vi "Query to Tree Information.vi"(7 "System or ALL Combined Fields":T1[](array[typedef]), 8 "error in (no error)":errorcluster, 9 "Load data? (t)":bool=TRUE, 10 "Load Fields? (f)":bool, 11 "Run Array":T9[](array[typedef])) -> (0 "error out":errorcluster, 1 "Total ms":u32, 3 "Data Tree":T4[](array[typedef]))   [LabVIEW 2011]
uses:
  www/cgi-bin/_cgi-lib/TDM_INDEX Record.ctl
  TDMS/TDMS Model Number.ctl
  TDMS/TDMS Serial Number.ctl
  TDMS/TDMS File.ctl
  TDMS/TDMS Run.ctl
  TDMS/TDMS Channel (Sxx).ctl
  database/Fields/Field Record.ctl
  database/Fields/Field DataTypes.ctl
  database/Fields/Field NextItem.ctl
panel:
  out "Time per file":dbl
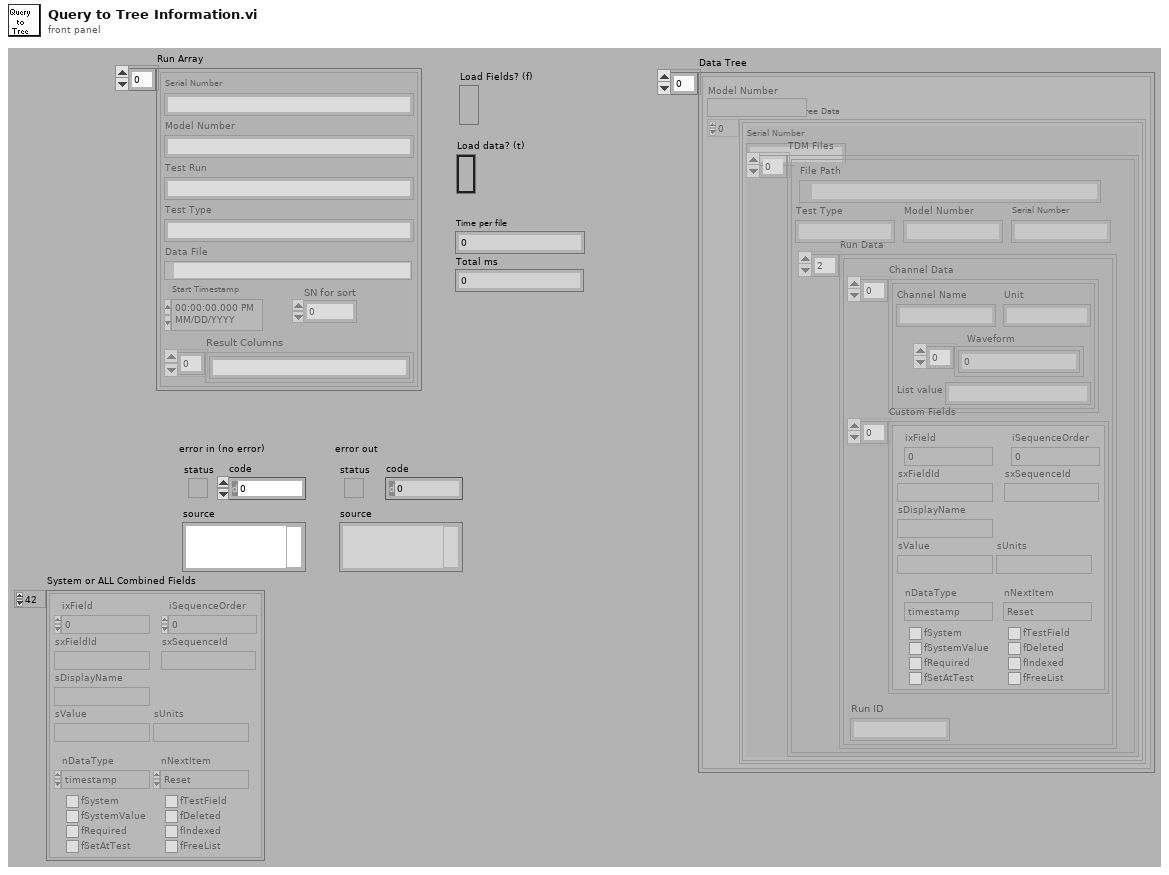
[diagram p1: front panel]
types:
  T1 = typedef "Field Record.ctl" = cluster{"ixField":i32, "iSequenceOrder":i32, "sxFieldId":string, "sxSequenceId":string, "sDisplayName":string, "sValue":string, "sUnits":string, "nDataType":T2, "nNextItem":T3, "fSystem":bool, "fSystemValue":bool, "fRequired":bool, "fSetAtTest":bool, "fTestField":bool, "fDeleted":bool, "fIndexed":bool, "fFreeList":bool}
  T2 = typedef "Field DataTypes.ctl" = enum32{"text", "numeric", "list", "timestamp", "boolean"}
  T3 = typedef "Field NextItem.ctl" = enum32{"Reset", "Retain", "Auto-Increment"}
  T4 = typedef "TDMS Model Number.ctl" = cluster{"Model Number":string, "Serial Number Tree Data":T5[]}
  T5 = typedef "TDMS Serial Number.ctl" = cluster{"Serial Number":string, "TDM Files":T6[]}
  T6 = typedef "TDMS File.ctl" = cluster{"File Path":path, "Run Data":T7[], "Serial Number":string, "Model Number":string, "Test Type":string}
  T7 = typedef "TDMS Run.ctl" = cluster{"Channel Data":T8[], "Custom Fields":T1[], "Run ID":string}
  T8 = typedef "TDMS Channel (Sxx).ctl" = cluster{"Channel Name":string, "Waveform":dbl[], "Unit":string, "List value":string}
  T9 = typedef "TDM_INDEX Record.ctl" = cluster{"Model Number":string, "SN for sort":i32, "Test Type":string, "Test Run":string, "Serial Number":string, "Start Timestamp":timestamp, "Data File":path, "Result Columns":string[]}
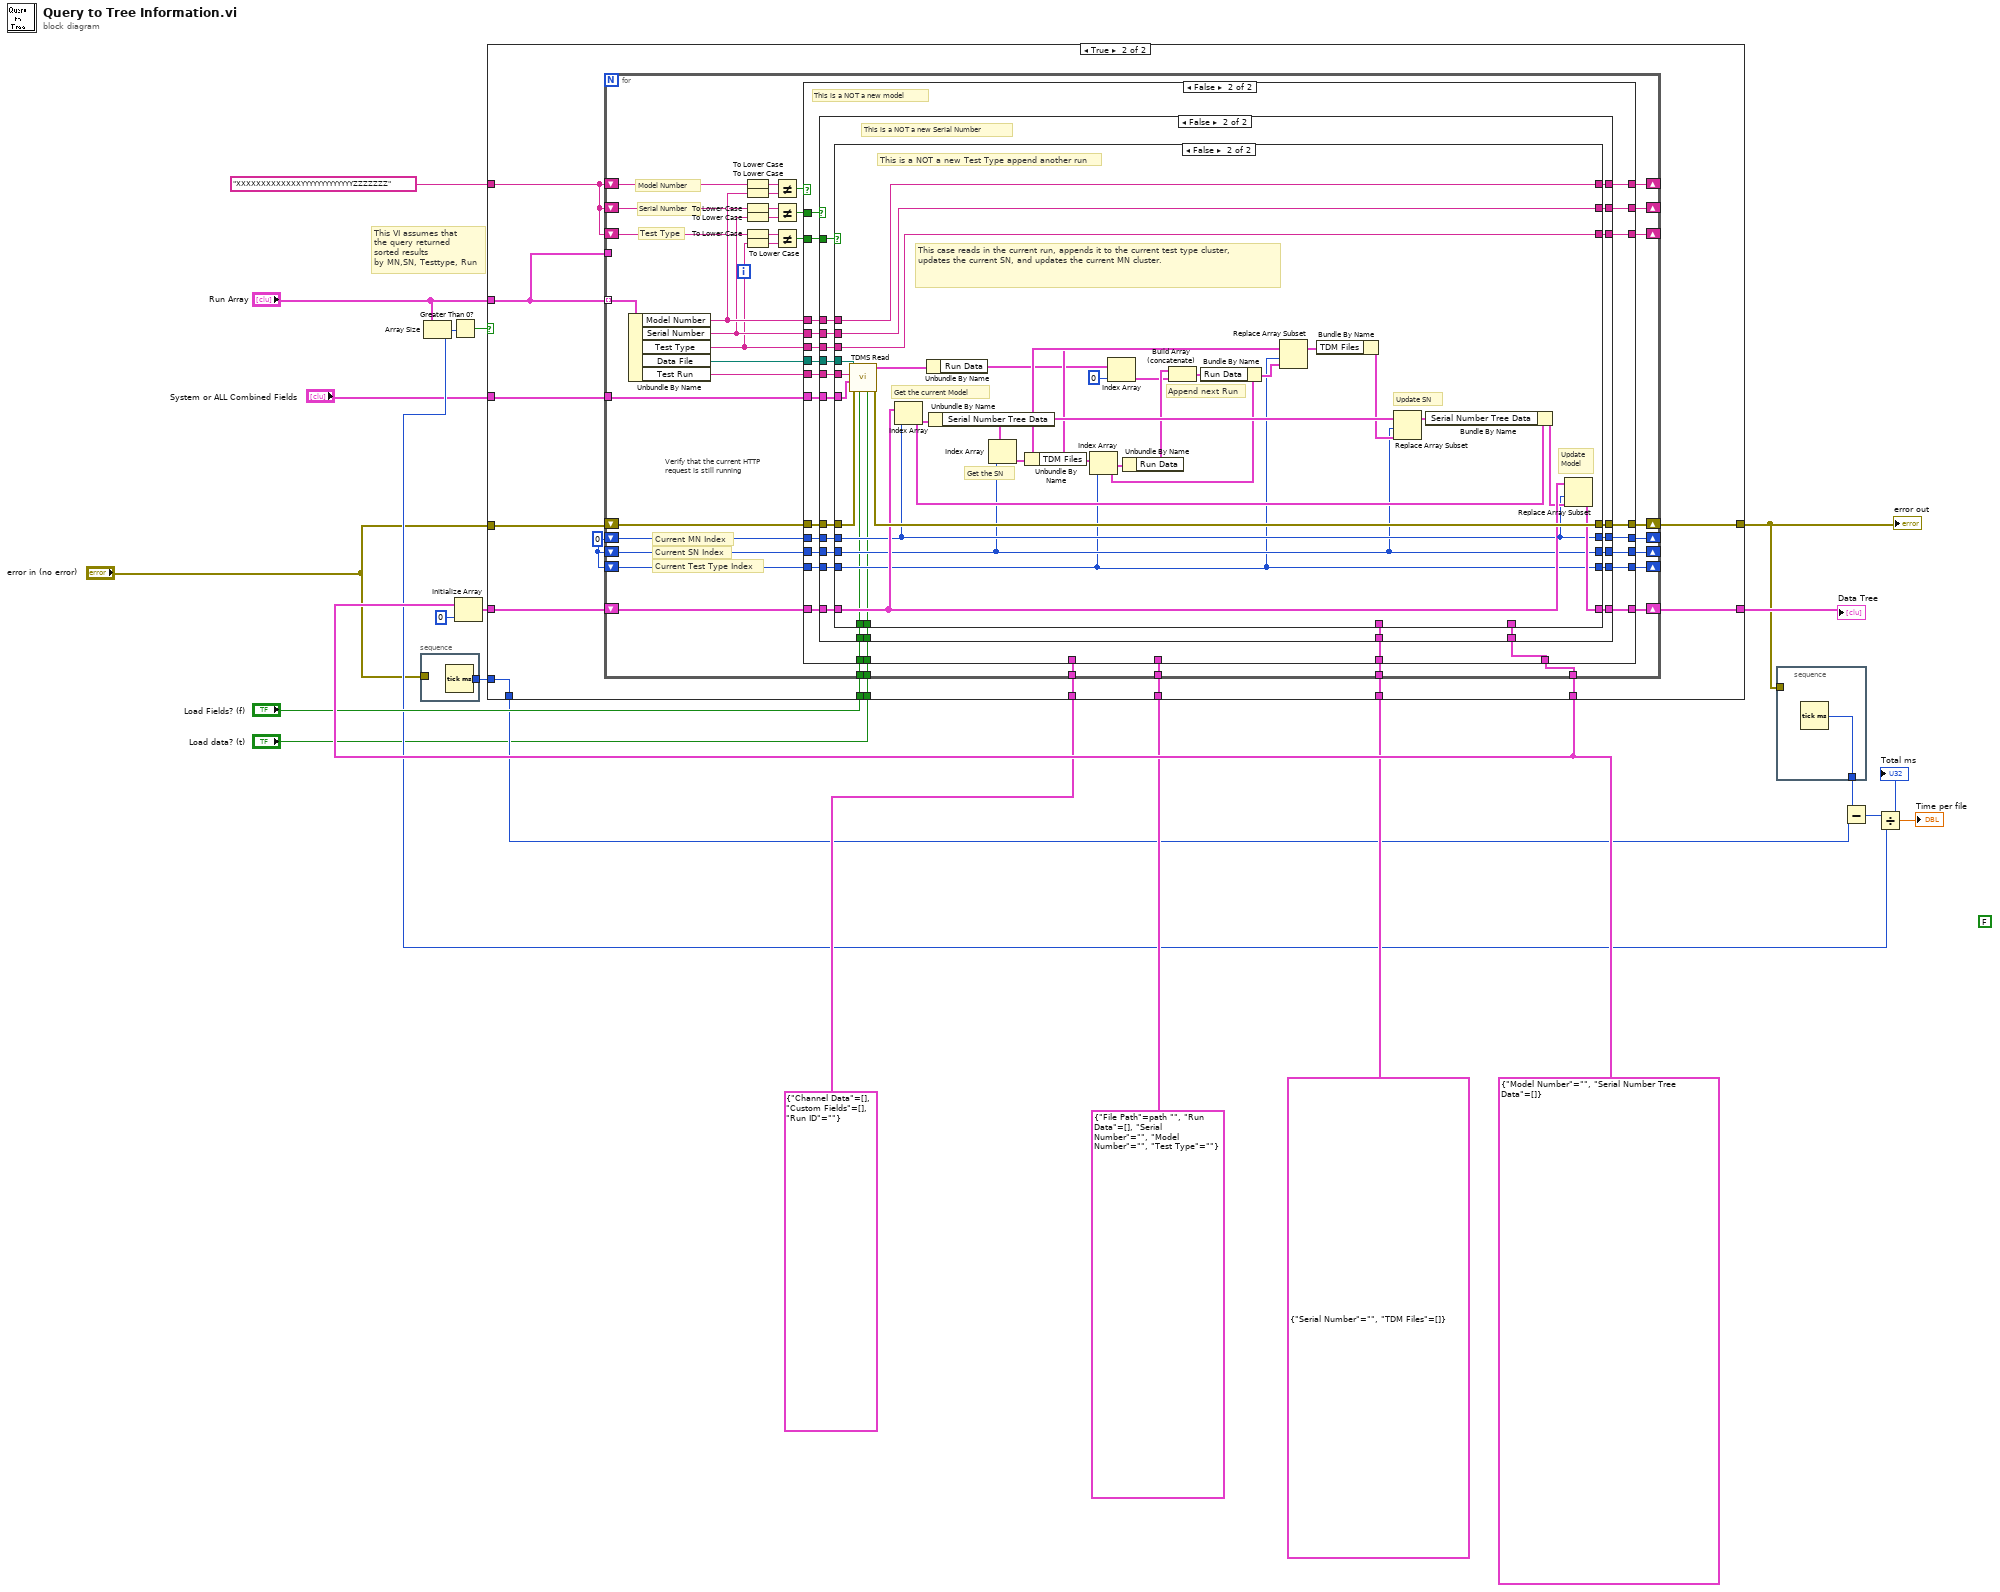
[diagram p0: block diagram]
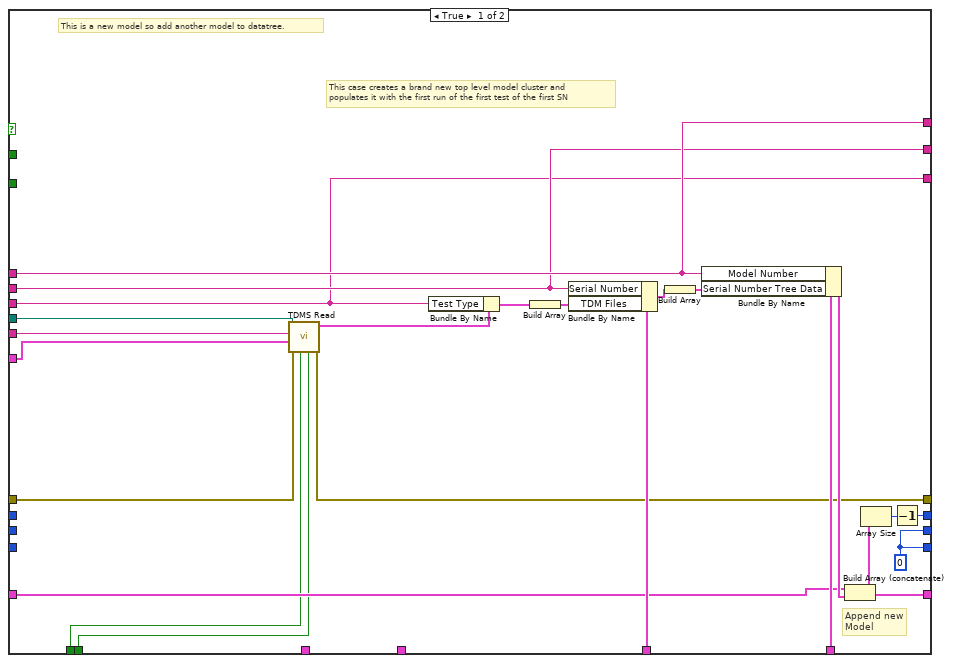
[diagram p3: hidden frame]
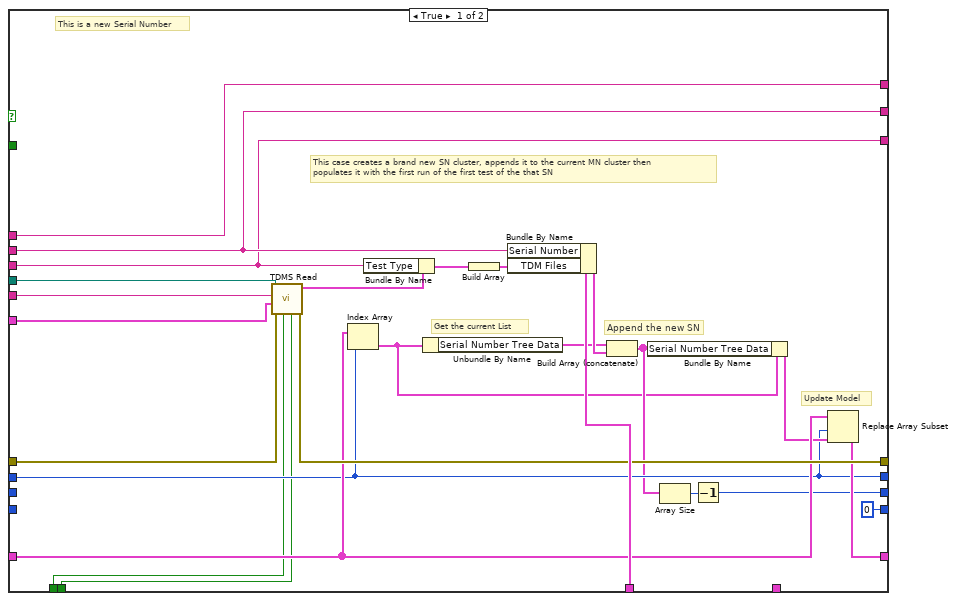
[diagram p4: hidden frame]
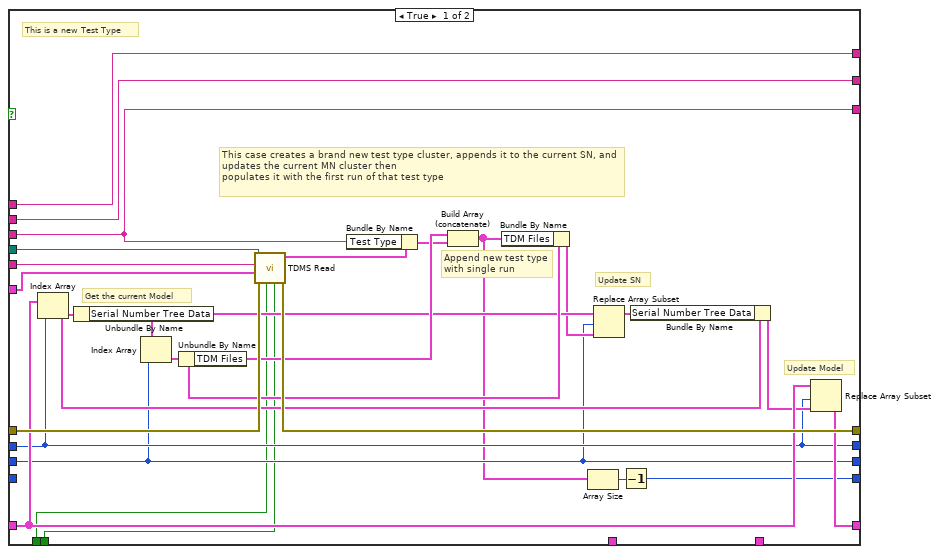
[diagram p5: hidden frame]
diagram:
  (unwired) FALSE
  w18 = T4 {"Model Number"="", "Serial Number Tree Data"=[]} ("Model Tree Data")
  # "This VI assumes that\nthe query returned\nsorted results\nby MN,SN, Testtype, Run"
  n1 = stacked-sequence {
    tunnel: [w22] -> w11
    tunnel: "error in (no error)" -> [_]
    frame #0 {
      n2 = Tick Count (ms)() -> (millisecond timer value=w22:u32)
    }
  }
  n3 = Array Size(array="Run Array") -> (size(s)=w9:i32)
  n4 = Greater Than 0?(x=w9) -> (x > 0?=w21:bool)
  n5 = Initialize Array(w18, 0 ("dimension size")) -> (w17:T4[])
  n6 = case shown="True" w21 {
    tunnel: "Run Array" -> [_ w28]
    tunnel: w18 -> [_ w39]
    tunnel: w17 -> [w25 w40]
    tunnel: [w25 w33] -> w7
    tunnel: T5 {"Serial Number"="", "TDM Files"=[]} ("Serial Number Data") -> [_ w38]
    tunnel: T6 {"File Path"=path "", "Run Data"=[], "Serial Number"="", "Model Number"="", "Test Type"=""} ("File Information") -> [_ w37]
    tunnel: T7 {"Channel Data"=[], "Custom Fields"=[], "Run ID"=""} ("Run Information") -> [_ w36]
    tunnel: "error in (no error)" -> [w24 w35]
    tunnel: [w24 w34] -> w5
    tunnel: "XXXXXXXXXXXXXYYYYYYYYYYYYYZZZZZZZ" -> [_ w31]
    tunnel: "Load Fields? (f)" -> [_ w30]
    tunnel: [w23 w29] -> w10
    tunnel: w11 -> [w23 w29]
    tunnel: "Load data? (t)" -> [_ w27]
    tunnel: "System or ALL Combined Fields" -> [_ w26]
    frame False {
      # "No Data"
    }
    frame True {
      w32 = 0
      n7 = for {
        tunnel: w28 -> [w78] mode=indexing
        shift-right: [w71] -> _
        shift-left: w31 -> [w77]
        shift-right: [w70] -> _
        shift-left: w31 -> [w62]
        shift-right: [w64] -> _
        shift-left: w31 -> [w53]
        shift-right: [w68] -> w33
        shift-left: w40 -> [w76]
        tunnel: w39 -> [w75]
        tunnel: w38 -> [w73]
        tunnel: w37 -> [w72]
        tunnel: w36 -> [w67]
        shift-right: [w65] -> w34
        shift-left: w35 -> [w43]
        shift-right: [w59] -> _
        shift-left: w32 -> [w60]
        shift-right: [w56] -> _
        shift-left: w32 -> [w58]
        shift-right: [w55] -> _
        shift-left: w32 -> [w57]
        tunnel: w30 -> [w44]
        tunnel: w28 -> [_]
        tunnel: w27 -> [w42]
        tunnel: w26 -> [w41]
        # "Verify that the current HTTP\nrequest is still running"
        # "Current Test Type Index"
        # "Current SN Index"
        # "Current MN Index"
        # "Test Type"
        # "Serial Number"
        # "Model Number"
        n8 = Unbundle By Name(w78) -> ("Model Number"=w74:string, "Serial Number"=w61:string, "Test Type"=w51:string, "Data File"=w69:path, "Test Run"=w66:string)
        n9 = To Lower Case(string=w77) -> (all lower case string=w50:string)
        n10 = To Lower Case(string=w74) -> (all lower case string=w49:string)
        n11 = To Lower Case(string=w62) -> (all lower case string=w48:string)
        n12 = To Lower Case(string=w61) -> (all lower case string=w47:string)
        n13 = To Lower Case(string=w53) -> (all lower case string=w46:string)
        n14 = To Lower Case(string=w51) -> (all lower case string=w45:string)
        n15 = Not Equal?(x=w50, y=w49) -> (x != y?=w63:bool)
        n16 = Not Equal?(x=w48, y=w47) -> (x != y?=w54:bool)
        n17 = Not Equal?(x=w46, y=w45) -> (x != y?=w52:bool)
        n18 = case shown="False" w63 {
          tunnel: w76 -> [w86 w118]
          tunnel: w75 -> [w101 w116]
          tunnel: w74 -> [w97 w114]
          tunnel: w73 -> [w100 w126]
          tunnel: w61 -> [w96 w125]
          tunnel: w72 -> [_ _]
          tunnel: [w97 w113] -> w71
          tunnel: [w96 w112] -> w70
          tunnel: w51 -> [w88 w121]
          tunnel: w69 -> [w93 w124]
          tunnel: [w83 w115] -> w68
          tunnel: w67 -> [_ _]
          tunnel: w66 -> [w87 w120]
          tunnel: w43 -> [w92 w123]
          tunnel: [w91 w122] -> w65
          tunnel: [w88 w111] -> w64
          tunnel: w60 -> [_ w117]
          tunnel: [w82 w110] -> w59
          tunnel: w54 -> [_ w119]
          tunnel: w58 -> [_ w109]
          tunnel: w57 -> [_ w108]
          tunnel: [w85 w107] -> w56
          tunnel: [w85 w106] -> w55
          tunnel: w52 -> [_ w105]
          tunnel: w44 -> [w81 w104]
          tunnel: w42 -> [w80 w103]
          tunnel: w41 -> [w79 w102]
          frame True {
            w85 = 0
            # "This case creates a brand new top level model cluster and \npopulates it with the first run of the first test of the first SN"
            # "This is a new model so add another model to datatree."
            # "Append new\nModel"
            n19 = call "TDMS Read.vi"("Load data?"=w80, "Load Fields?"=w81, "error in (no error)"=w92, "System or ALL Combined Fields"=w79, "Run String"=w87, "TDM File Path"=w93) -> ("error out"=w91:errorcluster, "File Information"=w90:T6)  [unwired: 2 in, 2 out]
            n20 = Bundle By Name(cluster=w90, "Test Type"=w88) -> (w89:T6)
            n21 = Build Array(w89) -> (w95:T6[])
            n22 = Bundle By Name(cluster=w100, "Serial Number"=w96, "TDM Files"=w95) -> (w99:T5)
            n23 = Build Array(w99) -> (w98:T5[])
            n24 = Bundle By Name(cluster=w101, "Model Number"=w97, "Serial Number Tree Data"=w98) -> (w94:T4)
            n25 = Build Array (concatenate)(w86, w94) -> (w83:T4[])
            n26 = Array Size(array=w83) -> (size(s)=w84:i32)
            n27 = Decrement(x=w84) -> (x-1=w82:i32)
          }
          frame False {
            # "This is a NOT a new model"
            n28 = case shown="False" w119 {
              tunnel: w126 -> [w151 w175]
              tunnel: w125 -> [w138 w165]
              tunnel: w124 -> [w149 w174]
              tunnel: w123 -> [w148 w173]
              tunnel: [w147 w172] -> w122
              tunnel: w121 -> [w137 w164]
              tunnel: w120 -> [w144 w171]
              tunnel: w118 -> [w142 w169]
              tunnel: w117 -> [w136 w170]
              tunnel: w116 -> [_ w168]
              tunnel: [w140 w167] -> w115
              tunnel: w114 -> [w139 w166]
              tunnel: [w139 w157] -> w113
              tunnel: [w138 w156] -> w112
              tunnel: [w137 w155] -> w111
              tunnel: [w136 w161] -> w110
              tunnel: w109 -> [_ w163]
              tunnel: w108 -> [_ w159]
              tunnel: [w131 w160] -> w107
              tunnel: [0 w158] -> w106
              tunnel: w105 -> [_ w162]
              tunnel: w104 -> [w129 w154]
              tunnel: w103 -> [w128 w153]
              tunnel: w102 -> [w127 w152]
              frame True {
                # "This case creates a brand new SN cluster, appends it to the current MN cluster then\npopulates it with the first run of the first test of the that SN"
                # "Update Model"
                # "Append the new SN"
                # "Get the current List"
                # "This is a new Serial Number"
                n29 = call "TDMS Read.vi"("Load data?"=w128, "Load Fields?"=w129, "error in (no error)"=w148, "System or ALL Combined Fields"=w127, "Run String"=w144, "TDM File Path"=w149) -> ("error out"=w147:errorcluster, "File Information"=w146:T6)  [unwired: 2 in, 2 out]
                n30 = Index Array(array=w142, index=w136) -> (element=w130:T4)
                n31 = Bundle By Name(cluster=w146, "Test Type"=w137) -> (w145:T6)
                n32 = Unbundle By Name(w130) -> ("Serial Number Tree Data"=w134:T5[])
                n33 = Build Array(w145) -> (w150:T6[])
                n34 = Bundle By Name(cluster=w151, "Serial Number"=w138, "TDM Files"=w150) -> (w143:T5)
                n35 = Build Array (concatenate)(w134, w143) -> (w133:T5[])
                n36 = Bundle By Name(cluster=w130, "Serial Number Tree Data"=w133) -> (w141:T4)
                n37 = Array Size(array=w133) -> (size(s)=w132:i32)
                n38 = Decrement(x=w132) -> (x-1=w131:i32)
                n39 = Replace Array Subset(array=w142, new element=w141, index=w136) -> (w140:T4[])
              }
              frame False {
                # "This is a NOT a new Serial Number"
                n40 = case shown="False" w162 {
                  tunnel: w175 -> [_ _]
                  tunnel: w174 -> [w201 w232]
                  tunnel: w173 -> [w200 w231]
                  tunnel: [w199 w230] -> w172
                  tunnel: w171 -> [w197 w229]
                  tunnel: w170 -> [w186 w220]
                  tunnel: w169 -> [w196 w228]
                  tunnel: w168 -> [_ _]
                  tunnel: [w194 w226] -> w167
                  tunnel: w166 -> [w184 w207]
                  tunnel: w165 -> [w183 w206]
                  tunnel: w164 -> [w182 w205]
                  tunnel: w163 -> [w185 w219]
                  tunnel: [w186 w220] -> w161
                  tunnel: [w185 w219] -> w160
                  tunnel: w159 -> [_ w208]
                  tunnel: [w179 w208] -> w158
                  tunnel: [w184 w207] -> w157
                  tunnel: [w183 w206] -> w156
                  tunnel: [w182 w205] -> w155
                  tunnel: w154 -> [w178 w204]
                  tunnel: w153 -> [w177 w203]
                  tunnel: w152 -> [w176 w202]
                  frame True {
                    # "This case creates a brand new test type cluster, appends it to the current SN, and updates the current MN cluster then\npopulates it with the first run of that test type"
                    # "Update SN"
                    # "Append new test type\nwith single run"
                    # "This is a new Test Type"
                    # "Update Model"
                    # "Get the current Model"
                    n41 = Index Array(array=w196, index=w186) -> (element=w187:T4)
                    n42 = Unbundle By Name(w187) -> ("Serial Number Tree Data"=w190:T5[])
                    n43 = Index Array(array=w190, index=w185) -> (element=w191:T5)
                    n44 = Unbundle By Name(w191) -> ("TDM Files"=w193:T6[])
                    n45 = call "TDMS Read.vi"("Load data?"=w177, "Load Fields?"=w178, "error in (no error)"=w200, "System or ALL Combined Fields"=w176, "Run String"=w197, "TDM File Path"=w201) -> ("error out"=w199:errorcluster, "File Information"=w198:T6)  [unwired: 2 in, 2 out]
                    n46 = Bundle By Name(cluster=w198, "Test Type"=w182) -> (w192:T6)
                    n47 = Build Array (concatenate)(w193, w192) -> (w180:T6[])
                    n48 = Bundle By Name(cluster=w191, "TDM Files"=w180) -> (w189:T5)
                    n49 = Array Size(array=w180) -> (size(s)=w181:i32)
                    n50 = Replace Array Subset(array=w190, new element=w189, index=w185) -> (w188:T5[])
                    n51 = Decrement(x=w181) -> (x-1=w179:i32)
                    n52 = Bundle By Name(cluster=w187, "Serial Number Tree Data"=w188) -> (w195:T4)
                    n53 = Replace Array Subset(array=w196, new element=w195, index=w186) -> (w194:T4[])
                  }
                  frame False {
                    # "This case reads in the current run, appends it to the current test type cluster, updates the current SN, and updates the current MN cluster."
                    # "Append next Run"
                    # "Get the SN"
                    # "Update SN"
                    # "This is a NOT a new Test Type append another run"
                    # "Update\nModel"
                    # "Get the current Model"
                    n54 = call "TDMS Read.vi"("Load data?"=w203, "Load Fields?"=w204, "error in (no error)"=w231, "System or ALL Combined Fields"=w202, "Run String"=w229, "TDM File Path"=w232) -> ("error out"=w230:errorcluster, "File Information"=w216:T6)  [unwired: 2 in, 2 out]
                    n55 = Index Array(array=w228, index=w220) -> (element=w221:T4)
                    n56 = Unbundle By Name(w216) -> ("Run Data"=w215:T7[])
                    n57 = Unbundle By Name(w221) -> ("Serial Number Tree Data"=w224:T5[])
                    n58 = Index Array(array=w224, index=w219) -> (element=w225:T5)
                    n59 = Unbundle By Name(w225) -> ("TDM Files"=w217:T6[])
                    n60 = Index Array(array=w217, index=w208) -> (element=w211:T6)
                    n61 = Index Array(array=w215, index=0) -> (element=w212:T7)
                    n62 = Unbundle By Name(w211) -> ("Run Data"=w213:T7[])
                    n63 = Build Array (concatenate)(w213, w212) -> (w209:T7[])
                    n64 = Bundle By Name(cluster=w211, "Run Data"=w209) -> (w210:T6)
                    n65 = Replace Array Subset(array=w217, new element=w210, index=w208) -> (w218:T6[])
                    n66 = Bundle By Name(cluster=w225, "TDM Files"=w218) -> (w223:T5)
                    n67 = Replace Array Subset(array=w224, new element=w223, index=w219) -> (w222:T5[])
                    n68 = Bundle By Name(cluster=w221, "Serial Number Tree Data"=w222) -> (w227:T4)
                    n69 = Replace Array Subset(array=w228, new element=w227, index=w220) -> (w226:T4[])
                  }
                }
              }
            }
          }
        }
      }
    }
  }
  "error out" <- w5
  "Data Tree" <- w7
  n70 = stacked-sequence {
    tunnel: [w233] -> w8
    tunnel: w5 -> [_]
    frame #0 {
      n71 = Tick Count (ms)() -> (millisecond timer value=w233:u32)
    }
  }
  n72 = Subtract(x=w8, y=w10) -> (x-y=w4:u32)
  "Total ms" <- w4
  n73 = Divide(x=w4, y=w9) -> (x/y=→"Time per file":dbl)
